vi "Send Assertion Update.vi"(8 "error in (no error)":errorcluster, 10 "Message":refnum<class "TestManagerMsg.lvclass">, 11 "Basic Test Manager in":refnum<class "Basic Test Manager.lvclass">) -> (0 "error out":errorcluster, 3 "Basic Test Manager out":refnum<class "Basic Test Manager.lvclass">)   [LabVIEW 2013, in "Caraya.lvlib" / "Basic Test Manager.lvclass"]
uses:
  Basic Test Manager.lvclass
  Test Manager Message/TestManagerMsg.lvclass
  MsgSerializer.JSON/MsgSerializer/MsgSerializer.JSON.lvclass
  Basic Test Manager.lvclass/Basic Test Manager.ctl
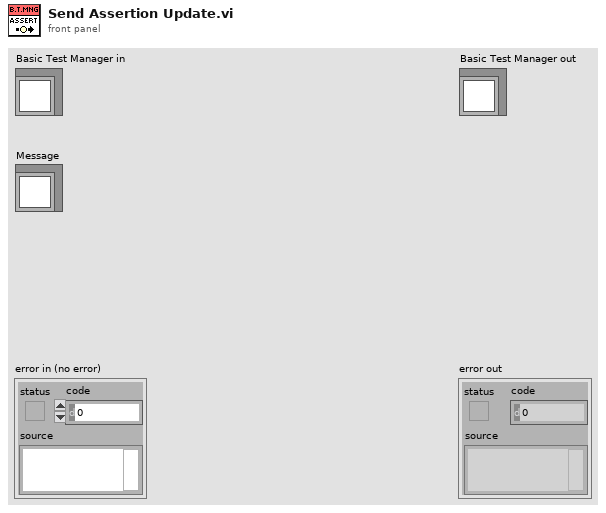
[diagram p1: front panel]
types:
  T1 = typedef "Caraya.lvlib/Test Result.lvclass/Test Events -- cluster.ctl" = cluster{"Test Registration Event":refnum<user-event>, "Assertion Event":refnum<user-event>, "Assertion Update Event":refnum<user-event>}
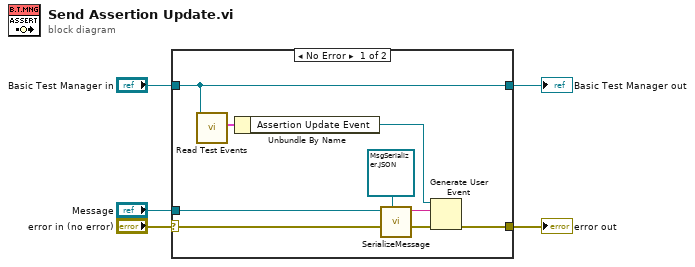
[diagram p0: block diagram]
diagram:
  n1 = case shown="No Error" "error in (no error)" {
    selector: "error in (no error)" -> [w7 w16]
    tunnel: [w6 w16] -> w4
    tunnel: [w9 w15] -> w2
    tunnel: "Basic Test Manager in" -> [w9 w15]
    tunnel: "Message" -> [w8 _]
    frame No Error {
      n2 = call "Read Test Events.vi"("Basic Test Manager in"=w9) -> ("Test Events"=w14:T1)  [unwired: 9 in, 1 out]
      n3 = Unbundle By Name(w14) -> ("Assertion Update Event"=w13:refnum<user-event>)
      n4 = call-dynamic "SerializeMessage.vi"("MsgSerializer"=refnum<class "MsgSerializer.JSON.lvclass"> refnum ("Caraya.lvlib:MsgSerializer.JSON.lvclass"), "error in (no error)"=w7, "TestManagerMsg in"=w8) -> ("error out"=w12:errorcluster, "Serialized Message"=w11:string)  [unwired: 7 in]
      n5 = Generate User Event(user event=w13, event data cluster=w11, error in=w12) -> (error out=w6:errorcluster)  [unwired: 1 in, 1 out]
    }
    frame Error {
    }
  }
  "error out" <- w4
  "Basic Test Manager out" <- w2
